vi "Final_gps.vi"() -> (0 "POSITION":string="BOT IS IN THE FARM", 1 "Distance to Destination m":dbl=920.0, 2 "Current Longitude [deg]":string="75.811895", 3 "Current Latitude [deg]":string="26.882130")   [LabVIEW 2013]
uses:
  <vilib>/Instr/_visa.llb/VISA Configure Serial Port (Instr).vi
panel:
  in  "To: 2":string="pankaj7897@outlook.com"
  out "Distance to Destination km":dbl=0.92
  in  "[ESC]":bool=TRUE
  out "NMEA sentences":string
  out "Time":string
  in  "time zone":i32
  out "UTC Time":string
  out "Latitude":string
  out "N/S":string
  out "Longitude":string
  out "E/W":string
  out "Speed over ground [knots]":string
  out "Status":string
  out "Course over ground [degrees]":string
  out "Date [ddmmyy]":string
  out "Mode":string
  in  "GPS PORT":refnum<visa-resource-name>="ASRL1::INSTR"
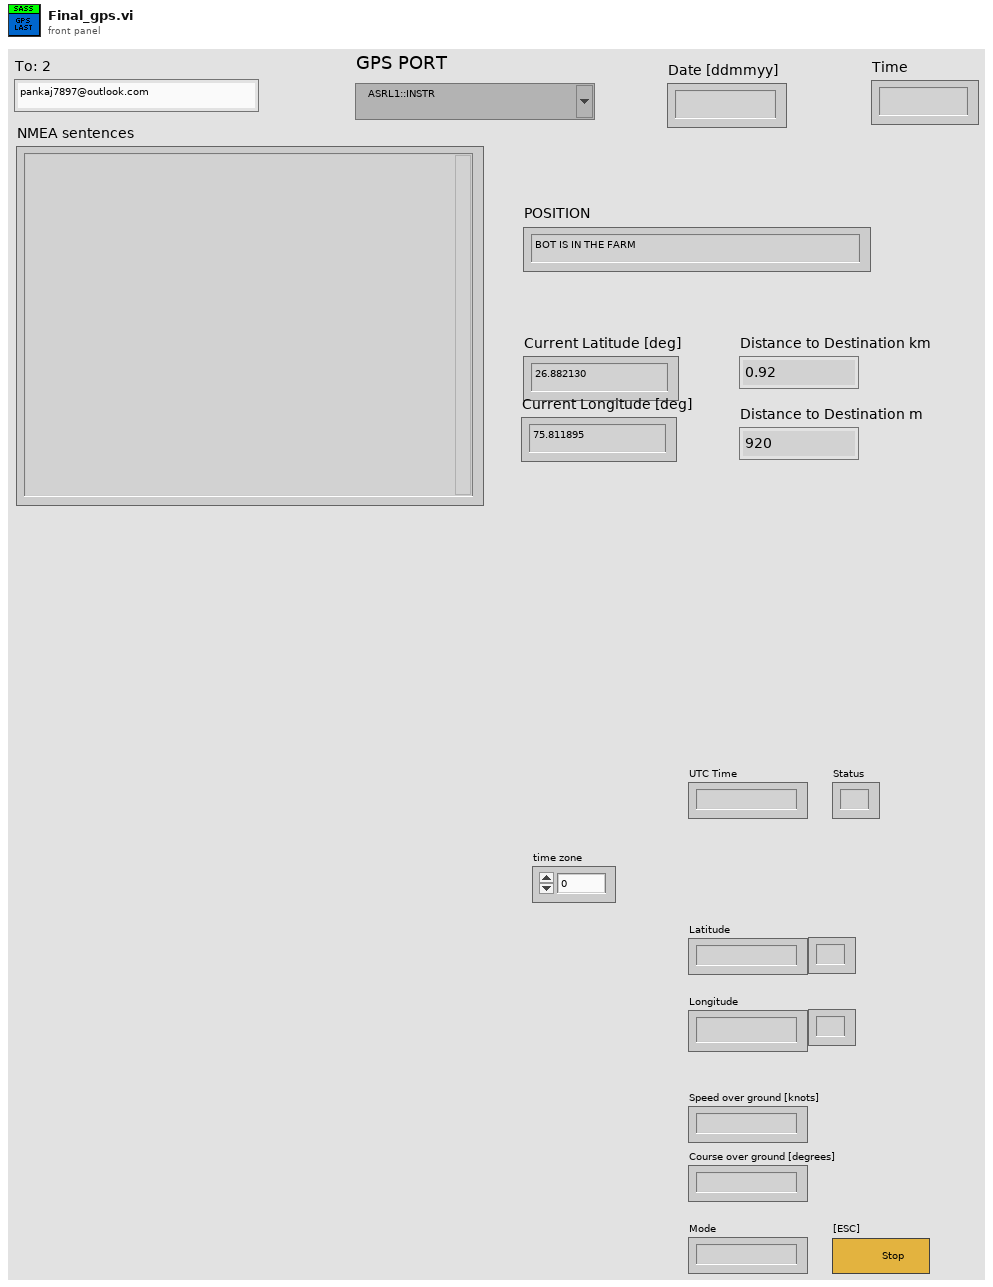
[diagram p1: front panel]
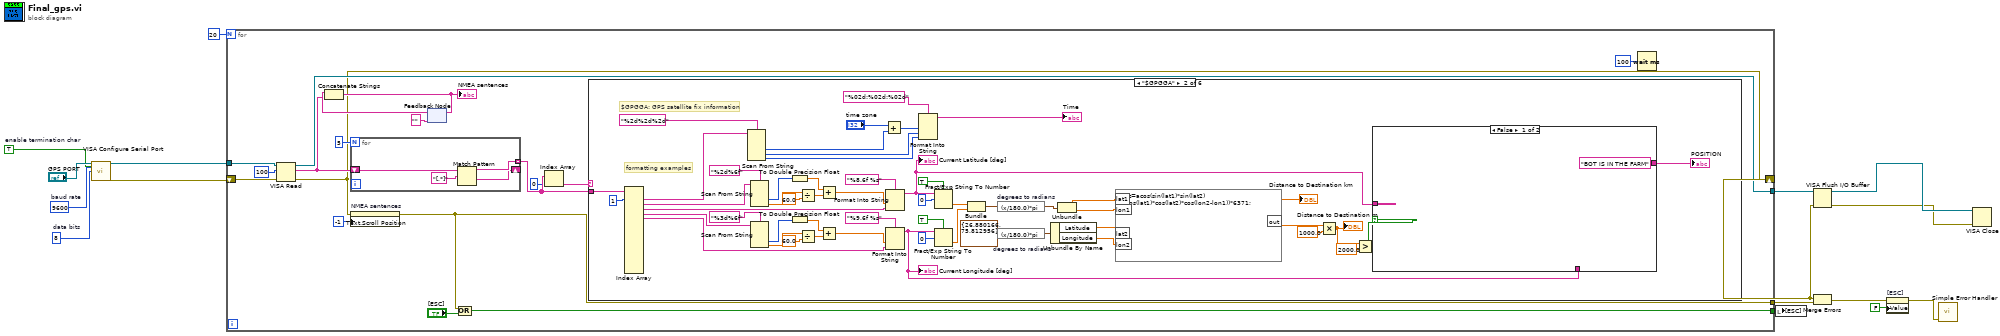
[diagram p0: block diagram]
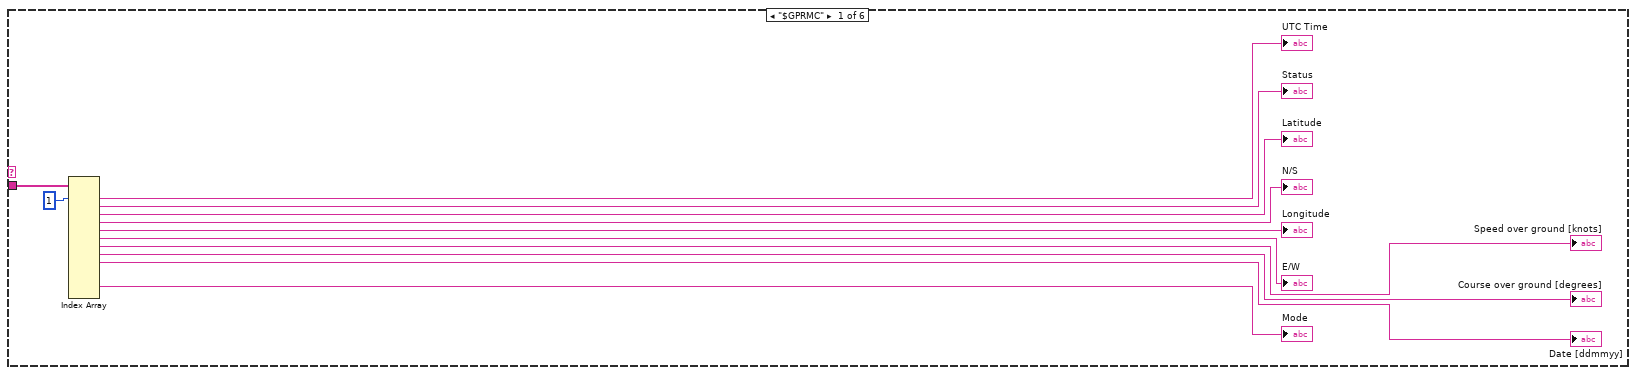
[diagram p2: hidden frame]
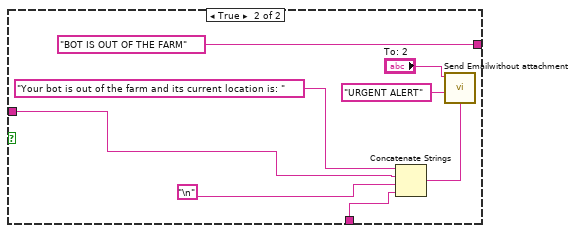
[diagram p3: hidden frame]
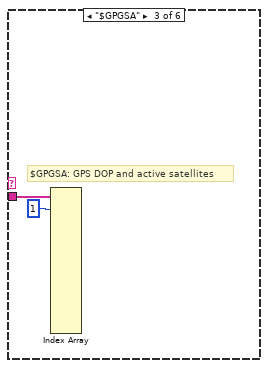
[diagram p4: hidden frame]
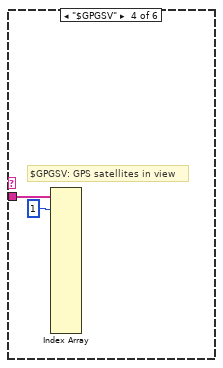
[diagram p5: hidden frame]
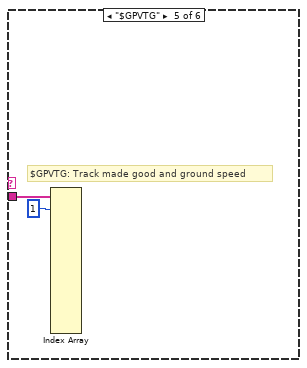
[diagram p6: hidden frame]
diagram:
  w11 = TRUE  # enable termination char
  w12 = u16 8  # data bits
  w13 = u32 9600  # baud rate
  n1 = call-poly "VISA Configure Serial Port"("VISA resource name"="GPS PORT", "Enable Termination\nChar (T)"=w11, "baud rate (9600)"=w13, "data bits (8)"=w12) -> ("VISA resource name out"=w14:refnum<visa-resource-name>, "error out"=w8:errorcluster)  [unwired: 10 in]
  n2 = for {
    N: 20 ("Numeric Control") -> [_]
    tunnel: [w22] -> w7
    tunnel: w14 -> [w32]
    tunnel: [w17] -> w6
    tunnel: [w20] -> w2
    shift-right: [w19] -> w1
    shift-left: w8 -> [w18]
    n3 = VISA Read(VISA resource name=w32, byte count=u32 100, error in (no error)=w18) -> (VISA resource name out=w20:refnum<visa-resource-name>, read buffer=w27:string, error out=w19:errorcluster)  [unwired: 1 out]
    n4 = for {
      N: 5 -> [_]
      tunnel: [w36] -> w25 mode=indexing
      shift-right: [w35] -> _
      shift-left: w27 -> [w37]
      n5 = Match Pattern(string=w37, regular expression="[,*]") -> (before substring=w36:string, after substring=w35:string)  [unwired: 1 in, 2 out]
    }
    n6 = property on="NMEA sentences" class="Str"(error in=w19, "Text.Scroll Position"=-1) -> (error out=w22:errorcluster)  [unwired: 1 in, 1 out]
    n7 = feedback #1("") -> (w29:string)
    n8 = Concatenate Strings "Concatenate Strings"(w29, w27) -> (w31:string)
    "NMEA sentences" <- w31
    n9 = feedback-in #1(w31) -> ()
    n10 = Or(x=w22, y="[ESC]") -> (x .or. y?=w17:bool)
    n11 = Index Array "Index Array"(array=w25, index=0) -> (element=w26:string)
    n12 = case shown="\"$GPGGA\"" w26 {
      tunnel: w25 -> [w50 w103 w114 w116 w118 _]
      frame "$GPRMC" {
        n13 = Index Array "Index Array"(array=w50, index #1=1 ("index")) -> (element #1=→"UTC Time":string, element #2=→"Status":string, element #3=→"Latitude":string, element #4=→"N/S":string, element #5=→"Longitude":string, element #6=→"E/W":string, element #7=→"Speed over ground [knots]":string, element #8=→"Course over ground [degrees]":string, element #9=→"Date [ddmmyy]":string, element #12=→"Mode":string)  [unwired: 12 in, 3 out]
      }
      frame "$GPGGA" {
        # "formatting examples"
        # "$GPGGA: GPS satellite fix information"
        n14 = Index Array "Index Array"(array=w103, index #1=1 ("index")) -> (element #1=w100:string, element #2=w91:string, element #3=w83:string, element #4=w74:string, element #5=w73:string)  [unwired: 15 in, 11 out]
        n15 = Scan From String "Scan From String"(format string="%2d%2d%2d", input string=w100) -> (output 1=w93:i32, output 2=w96:i32, output 3=w98:i32)  [unwired: 5 in, 3 out]
        n16 = Scan From String(format string="%2d%6f", input string=w91) -> (output 1=w88:i32, output 2=w90:dbl)  [unwired: 4 in, 3 out]
        n17 = Scan From String(format string="%3d%6f", input string=w74) -> (output 1=w78:i32, output 2=w76:dbl)  [unwired: 4 in, 3 out]
        n18 = To Double Precision Float(number=w88) -> (double precision float=w86:dbl)
        n19 = To Double Precision Float(number=w78) -> (double precision float=w80:dbl)
        n20 = Divide(x=w90, y=60.0) -> (x/y=w87:dbl)
        n21 = Divide(x=w76, y=60.0) -> (x/y=w79:dbl)
        n22 = Add(x=w86, y=w87) -> (x+y=w84:dbl)
        n23 = Add(x=w80, y=w79) -> (x+y=w82:dbl)
        n24 = Add(x="time zone", y=w93) -> (x+y=w94:i32)
        n25 = Format Into String(format string="%8.6f %s", w84, w83) -> (resulting string=w52:string)  [unwired: 2 in, 1 out]
        "Current Latitude [deg]" <- w52
        n26 = Format Into String(format string="%9.6f %s", w82, w73) -> (resulting string=w54:string)  [unwired: 2 in, 1 out]
        "Current Longitude [deg]" <- w54
        n27 = Format Into String "Format Into String"(format string="%02d:%02d:%02d", w94, w96, w98) -> (resulting string=→"Time":string)  [unwired: 2 in, 1 out]
        n28 = Fract/Exp String To Number(use system decimal point (T)=TRUE ("Systemdezimalzeichen verwenden (T)"), string=w52, offset=0) -> (number=w62:dbl)  [unwired: 1 in, 1 out]
        n29 = Fract/Exp String To Number(use system decimal point (T)=TRUE ("Systemdezimalzeichen verwenden (T)"), string=w54, offset=0) -> (number=w61:dbl)  [unwired: 1 in, 1 out]
        n30 = Bundle(w62, w61) -> (w60:cluster{dbl, dbl})  [unwired: 1 in]
        n31 = expression code="(x/180.0)*pi" "degrees to radians"(w60) -> (w59:cluster{dbl, dbl})
        n32 = expression code="(x/180.0)*pi" "degrees to radians"(cluster{"Latitude":dbl, "Longitude":dbl} {"Latitude"=26.880166, "Longitude"=75.812956} ("Current Location (degrees)")) -> (w68:cluster{"Latitude":dbl, "Longitude":dbl})
        n33 = Unbundle By Name(w68) -> ("Latitude"=w72:dbl, "Longitude"=w71:dbl)
        n34 = Unbundle(w59) -> (w58:dbl, w57:dbl)
        n35 = formula code="out=acos(sin(lat1)*sin(lat2)\n+cos(lat1)*cos(lat2)*cos(lon2-lon1))*6371;"("lat1"=w58, "lat2"=w72, "lon1"=w57, "lon2"=w71) -> ("out"=w70:dbl)
        "Distance to Destination km" <- w70
        n36 = Multiply(x=w70, y=1000.0) -> (x*y=w56:dbl)
        "Distance to Destination m" <- w56
        n37 = Greater?(x=w56, y=2000.0) -> (0:w53:bool)
        n38 = case shown="False" w53 {
          tunnel: w52 -> [_ w107]
          tunnel: w54 -> [_ w105]
          tunnel: ["BOT IS IN THE FARM" ("String") "BOT IS OUT OF THE FARM" ("String")] -> w51
          frame False {
          }
          frame True {
            n39 = Concatenate Strings("Your bot is out of the farm and its current location is: " ("string"), w107, "\n", w105) -> (w111:string)
            n40 = call "Send Emailwithout attachment.vi"("To: 2"="To: 2", "Subject 2"="URGENT ALERT", "Message 2"=w111) -> ()  [unwired: 8 in]
          }
        }
        "POSITION" <- w51
      }
      frame "$GPGSA" {
        # "$GPGSA: GPS DOP and active satellites"
        n41 = Index Array(array=w114, index #1=1 ("index")) -> ()  [unwired: 15 in, 16 out]
      }
      frame "$GPGSV" {
        # "$GPGSV: GPS satellites in view"
        n42 = Index Array(array=w116, index #1=1 ("index")) -> ()  [unwired: 15 in, 16 out]
      }
      frame "$GPVTG" {
        # "$GPVTG: Track made good and ground speed"
        n43 = Index Array(array=w118, index #1=1 ("index")) -> ()  [unwired: 15 in, 16 out]
      }
      frame Default {
      }
    }
    n44 = Wait (ms)(milliseconds to wait=u32 100) -> ()  [unwired: 1 out]
  }
  n45 = local write "[ESC]"(w6) -> ()
  n46 = VISA Flush I/O Buffer(VISA resource name=w2, error in (no error)=w1) -> (VISA resource name out=w10:refnum<visa-resource-name>, error out=w9:errorcluster)  [unwired: 1 in]
  n47 = Merge Errors "Merge Errors"(w1, w7) -> (w4:errorcluster)
  n48 = property on="[ESC]" class="Bool (strict)"(error in=w4, "Value"=FALSE ("[ESC]")) -> (error out=w16:errorcluster)  [unwired: 1 in, 1 out]
  n49 = call <vilib>:"Simple Error Handler.vi"("error in (no error)"=w16) -> ()  [unwired: 4 in, 5 out]
  n50 = VISA Close(VISA resource name=w10, error in (no error)=w9) -> ()  [unwired: 1 out]
